vi "String Parser.vi"(10 "Raw String":string) -> (2 "Value":dbl)   [LabVIEW 2020]
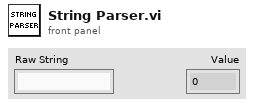
[diagram p1: front panel]
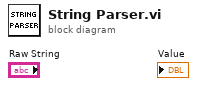
[diagram p0: block diagram]
diagram:
